vi "MyG#G3Templ_GetClassAttributes.vi"(0 "reference in":refnum<class "MyG#G3Templ.lvclass">, 1 "return data":bool=TRUE, 5 "error in (no error)":errorcluster) -> (14 "reference out":refnum<class "MyG#G3Templ.lvclass">, 15 "class attributes ref":T2, 16 "class attributes":T1, 17 "created new":bool, 19 "error out":errorcluster)   [LabVIEW 2017, in "MyG#G3Templ.lvclass"]
doc: "Returns a reference and if wanted the actual data values of the class attributes. This method is used by the subclasses to access parent class attributes."
uses:
  MyG#G3Templ.lvclass
  ClassAttributesRef.ctl
  protected/ClassAttributes.ctl
  C:/Program Files/National Instruments/LabVIEW 2017/vi.lib/addons/_AddQ/G#Object/G#Object.lvclass
  <vilib>/addons/_AddQ/G#Object/G#Object.lvclass
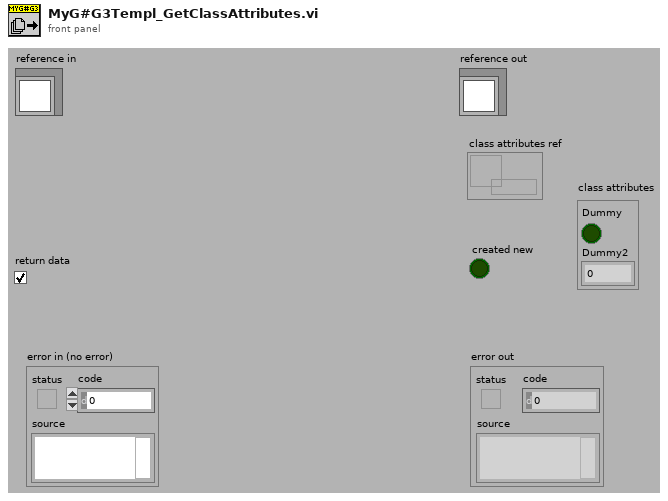
[diagram p1: front panel]
types:
  T1 = typedef "MyG#G3Templ.lvclass/ClassAttributes.ctl" = cluster{"Dummy":bool, "Dummy2":dbl}
  T2 = typedef "MyG#G3Templ.lvclass/ClassAttributesRef.ctl" = refnum<data-value>
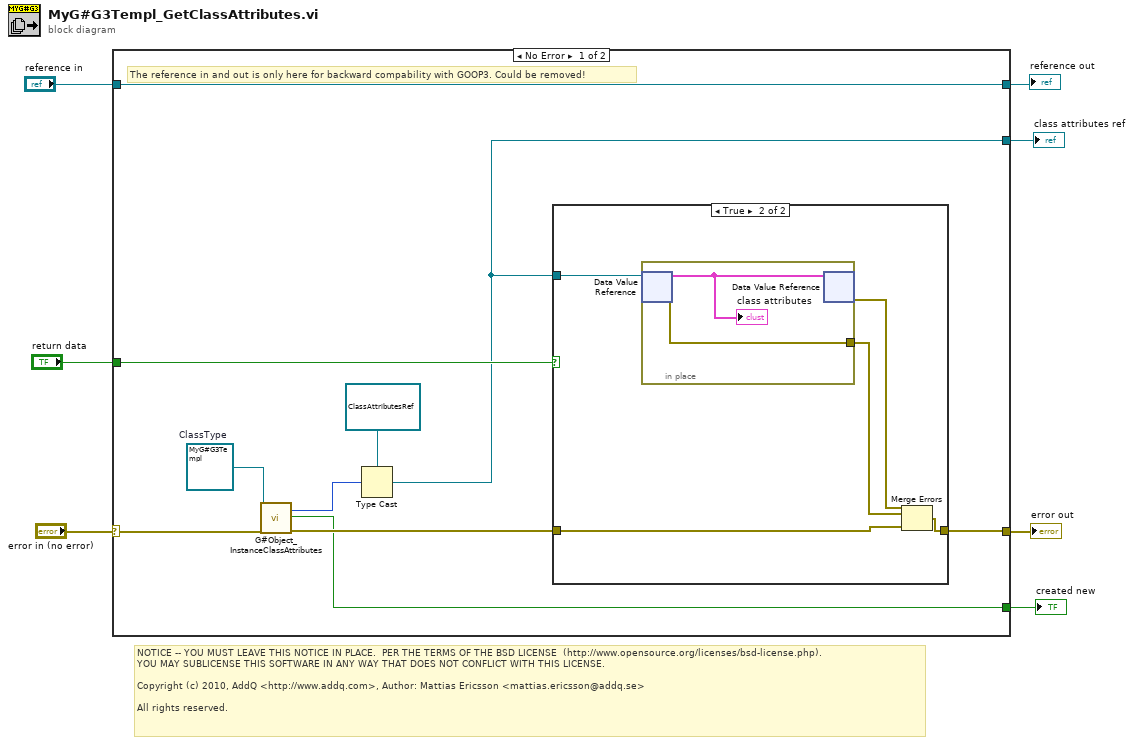
[diagram p0: block diagram]
diagram:
  # "NOTICE -- YOU MUST LEAVE THIS NOTICE IN PLACE.  PER THE TERMS OF THE BSD LICENSE  (http://www.opensource.org/licenses/bsd-license.php).\nYOU MAY SUBLICENSE THIS SOFTWARE IN ANY WAY THAT DOES NOT CONFLICT WITH THIS LICENSE.\n\nCopyright (c) 2010, AddQ <http://www.addq.com>, Author: Mattias Ericsson <mattias.ericsson@addq.se>\n\nAll rights reserved."
  n1 = case shown="No Error" "error in (no error)" {
    selector: "error in (no error)" -> [w12 w27]
    tunnel: [w17 w27] -> w6
    tunnel: [w14 _] -> w5
    tunnel: "return data" -> [w16 _]
    tunnel: "reference in" -> [w13 w26]
    tunnel: [w13 w26] -> w2
    tunnel: [w8 _] -> w1
    frame No Error {
      w10 = refnum<class "MyG#G3Templ.lvclass"> refnum  # ClassType
      # "The reference in and out is only here for backward compability with GOOP3. Could be removed!"
      n2 = call <vilib>:"G#Object_InstanceClassAttributes.vi"("reference in"=w10, "error in (no error)"=w12) -> ("static attribute ref"=w9:u32, "created new?"=w8:bool, "error out"=w11:errorcluster)  [unwired: 14 in, 1 out]
      n3 = Type Cast(type=T2 refnum ("data value reference"), x=w9) -> (*(type *) &x=w14:T2)
      n4 = case shown="True" w16 {
        tunnel: w11 -> [w18 w21]
        tunnel: [w18 w22] -> w17
        tunnel: w14 -> [_ w23]
        frame False {
        }
        frame True {
          n5 = in-place {
            in-place-border: [w25] -> w19
            n6 = in-place-dvr #1(w23) -> (w24:T1, w25:errorcluster)
            "class attributes" <- w24
            n7 = in-place-dvr #1(w24) -> (w20:errorcluster)  [unwired: 1 out]
          }
          n8 = Merge Errors(w20, w19, w21) -> (w22:errorcluster)
        }
      }
    }
    frame Error {
    }
  }
  "error out" <- w6
  "class attributes ref" <- w5
  "reference out" <- w2
  "created new" <- w1
